vi "get_freq_vector.vi"(11 "FFT magnitude":cluster{"f0":dbl, "df":dbl, "magnitude":dbl[]}) -> (3 "Freq array":dbl[](array[numeric]))   [LabVIEW 2021]
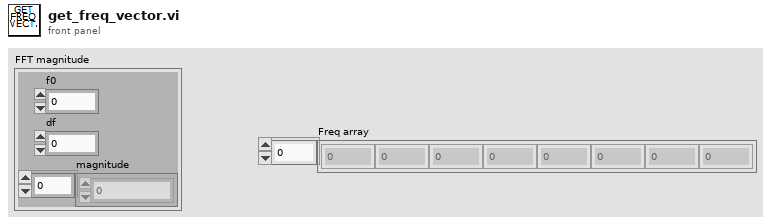
[diagram p1: front panel]
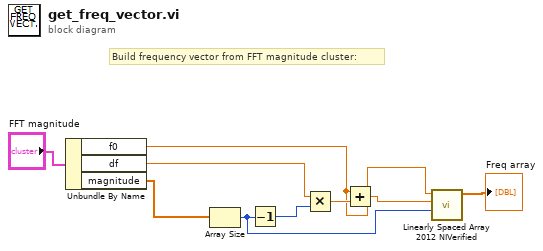
[diagram p0: block diagram]
diagram:
  # "Build frequency vector from FFT magnitude cluster:"
  n1 = Unbundle By Name("FFT magnitude") -> ("f0"=w1:dbl, "df"=w2:dbl, "magnitude"=w3:dbl[])
  n2 = Array Size(array=w3) -> (size(s)=w6:i32)
  n3 = Decrement(x=w6) -> (x-1=w8:i32)
  n4 = Multiply(x=w2, y=w8) -> (x*y=w9:dbl)
  n5 = Add(x=w1, y=w9) -> (x+y=w7:dbl)
  n6 = call "Linearly Spaced Array 2012 NIVerified.vi"("Number of Samples"=w6, "Maximum"=w7, "Minimum"=w1) -> ("Array"=→"Freq array":dbl[])  [unwired: 7 in, 1 out]
